vi "Init.vi"(8 "error in (no error)":errorcluster, 11 "Thermometer DAQmx Base CFG in":refnum<class "Thermometer DAQmx Base CFG.lvclass">) -> (0 "error out":errorcluster, 3 "Thermometer DAQmx Base CFG out":refnum<class "Thermometer DAQmx Base CFG.lvclass">)   [LabVIEW 2023, in "Thermometer DAQmx Base CFG.lvlib" / "Thermometer DAQmx Base CFG.lvclass"]
uses:
  Thermometer DAQmx Base CFG.lvclass
  <vilib>/Utility/error.llb/Error Cluster From Error Code.vi
  <vilib>/ErrorRing/Error Ring.xnode
  Thermometer DAQmx Base CFG.lvclass/Thermometer DAQmx Base CFG.ctl
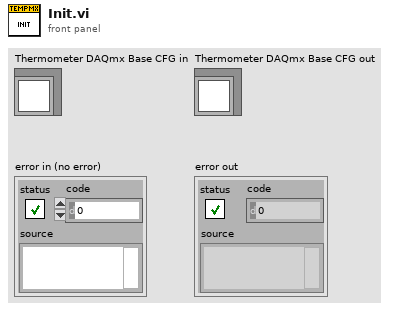
[diagram p1: front panel]
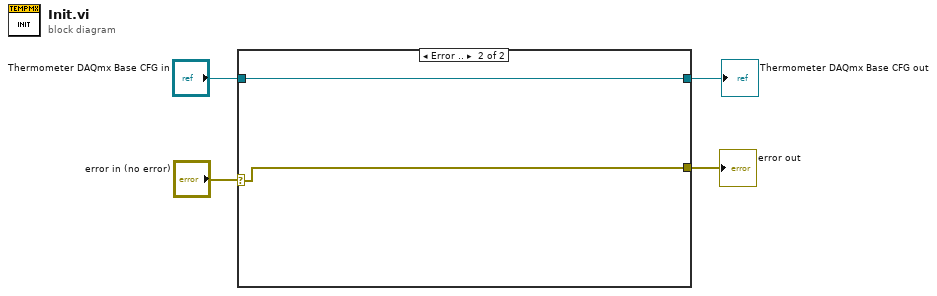
[diagram p0: block diagram]
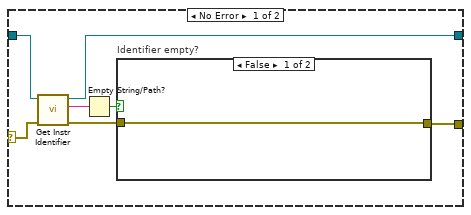
[diagram p2: hidden frame]
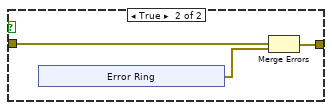
[diagram p3: hidden frame]
diagram:
  n1 = case shown="Error .." "error in (no error)" {
    selector: "error in (no error)" -> [w11 w21]
    tunnel: "Thermometer DAQmx Base CFG in" -> [w10 w22]
    tunnel: [w9 w22] -> w3
    tunnel: [w5 w21] -> w1
    frame No Error {
      n2 = call-dynamic "Get Instr Identifier.vi"("error in (no error)"=w11, "Configuration Base in"=w10) -> ("error out"=w6:errorcluster, "Instr Identifier"=w8:string, "Configuration Base out"=w9:refnum<class "Thermometer DAQmx Base CFG.lvclass">)  [unwired: 7 in]
      n3 = Empty String/Path?(string/path=w8) -> (empty?=w7:bool)
      n4 = case "Identifier empty?" shown="False" w7 {
        tunnel: w6 -> [w12 w15]
        tunnel: [w12 w14] -> w5
        frame False {
        }
        frame True {
          n5 = xnode "Error Ring"() -> ("error out"=w13:errorcluster)
          n6 = Merge Errors(w15, w13) -> (w14:errorcluster)
        }
      }
    }
    frame Error {
    }
  }
  "error out" <- w1
  "Thermometer DAQmx Base CFG out" <- w3
